vi "Close.vi"(8 "error in (no error)":errorcluster, 11 "HTTPHeaders_NET in":refnum<class "HttpHeaders_NET.lvclass">) -> (0 "error out":errorcluster)   [LabVIEW 2018, in "HttpClient_NET.lvlib" / "HttpHeaders_NET.lvclass"]
doc: "<b> </b> <b> </b>\nHttpClient_NET\nJustin Young - Viviota\nCopyright (c) 2021\nLicense: BSD"
uses:
  HttpHeaders_NET.lvclass
  HttpHeaders_NET.lvclass/HttpHeaders_NET.ctl
  Accessors/Read NET_HttpHeaders.vi
  System.Net.Http
panel:
  out "reference out":refnum<class "HttpHeaders_NET.lvclass">
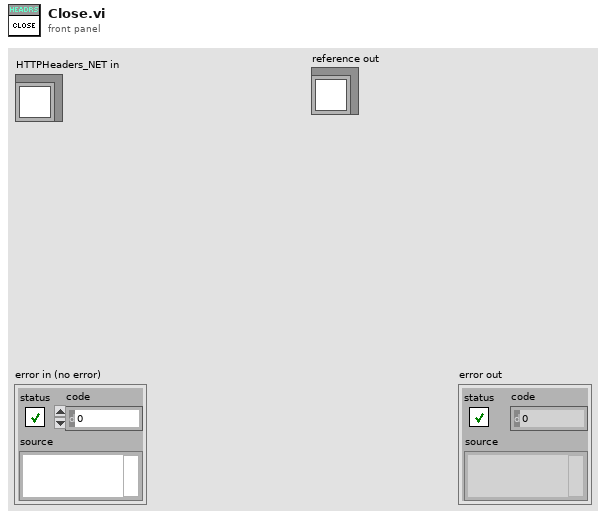
[diagram p1: front panel]
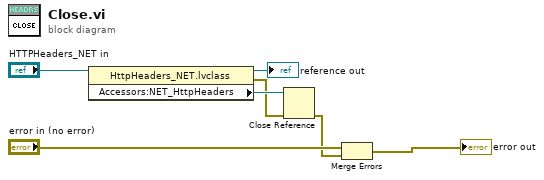
[diagram p0: block diagram]
diagram:
  n1 = property class="HttpHeaders_NET.lvclass"(reference="HTTPHeaders_NET in") -> (reference out=→"reference out":refnum<class "HttpHeaders_NET.lvclass">, error out=w4:errorcluster, "Accessors:NET_HttpHeaders"=w5:refnum<k24>)  [unwired: 1 in]
  n2 = Close Reference(reference=w5, error in (no error)=w4) -> (error out=w2:errorcluster)
  n3 = Merge Errors("error in (no error)", w2) -> (→"error out":errorcluster)
